vi "Input_Shared_Variable.vi"() -> (0 "Shared Variable Out":refnum<k21>)   [LabVIEW 2016]
panel:
  in  "Continue":bool
  in  "New Variable":refnum<k21>
  # "Input your new variable here:"
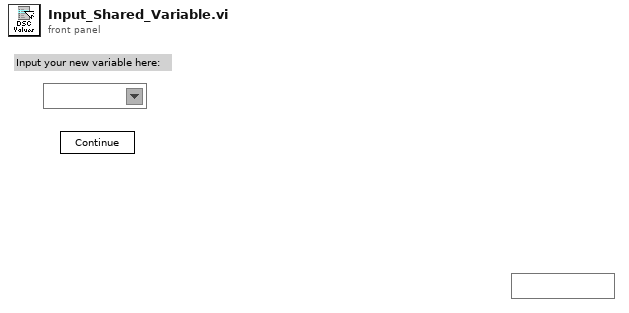
[diagram p1: front panel]
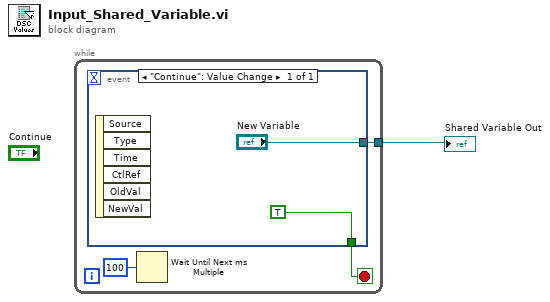
[diagram p0: block diagram]
diagram:
  n1 = while {
    tunnel: [w2] -> w1
    stop <- w4 stop-if-true
    n2 = event shown="[0] \"Continue\": Value Change" {
      selector: _ -> [_]
      dyn-events: _ -> [_]
      timeout: _ -> [_]
      tunnel: [TRUE] -> w4
      tunnel: ["New Variable"] -> w2
      event "Continue": Value Change {
        n3 = event-data() -> ()  [unwired: 1 in, 6 out]
      }
    }
    n4 = Wait Until Next ms Multiple(millisecond multiple=u32 100) -> ()  [unwired: 1 out]
  }
  "Shared Variable Out" <- w1
